vi "draw_spawn_positions.vi"(4 "error in":errorcluster, 7 "simx in":T1) -> (0 "error out":errorcluster, 3 "simx out":T1={"Config"={"Trajectory"={"Number of frames"=0, "Frame number"=0, "Trajectory"=""}, "Weather"={"id"=""}}, "Connections"={"Simulator Connection"=refnum, "server_ip"="127.0.0.1", "Port"=0, "Sensor connections"=[]}, "Map"={"lanes"={"x"=[], "y"=[], "z"=[]}, "StartPosition"={"start_points"={"locations"=[], "rotations"=[], "type"=[]}, "StartRotation"=[], "StartLocation"=[]}, "Draw Map Size"={"Width"=0, "Height"=0}, "DrawArea"={"min_Y"=0.0, "min_X"=0.0, "Scale X"=0.0, "Scale Y"=0.0}, "Map"=bytes[0], "Map Geojson"=""}})   [LabVIEW 2025]
doc: "Draw the possible spawn positions for the EGO vehicle on the map as dots. Adds the string \"Camera\" for the position where the camera is pointing (only on Editor mode)."
uses:
  controls/simx_connection.ctl
  controls/config.ctl
  controls/trajectory.ctl
  controls/weather.ctl
  controls/connections.ctl
  controls/start_points.ctl
  <vilib>/Utility/miscctls.llb/LVBoundsTypeDef.ctl
panel:
  out "Map":picture
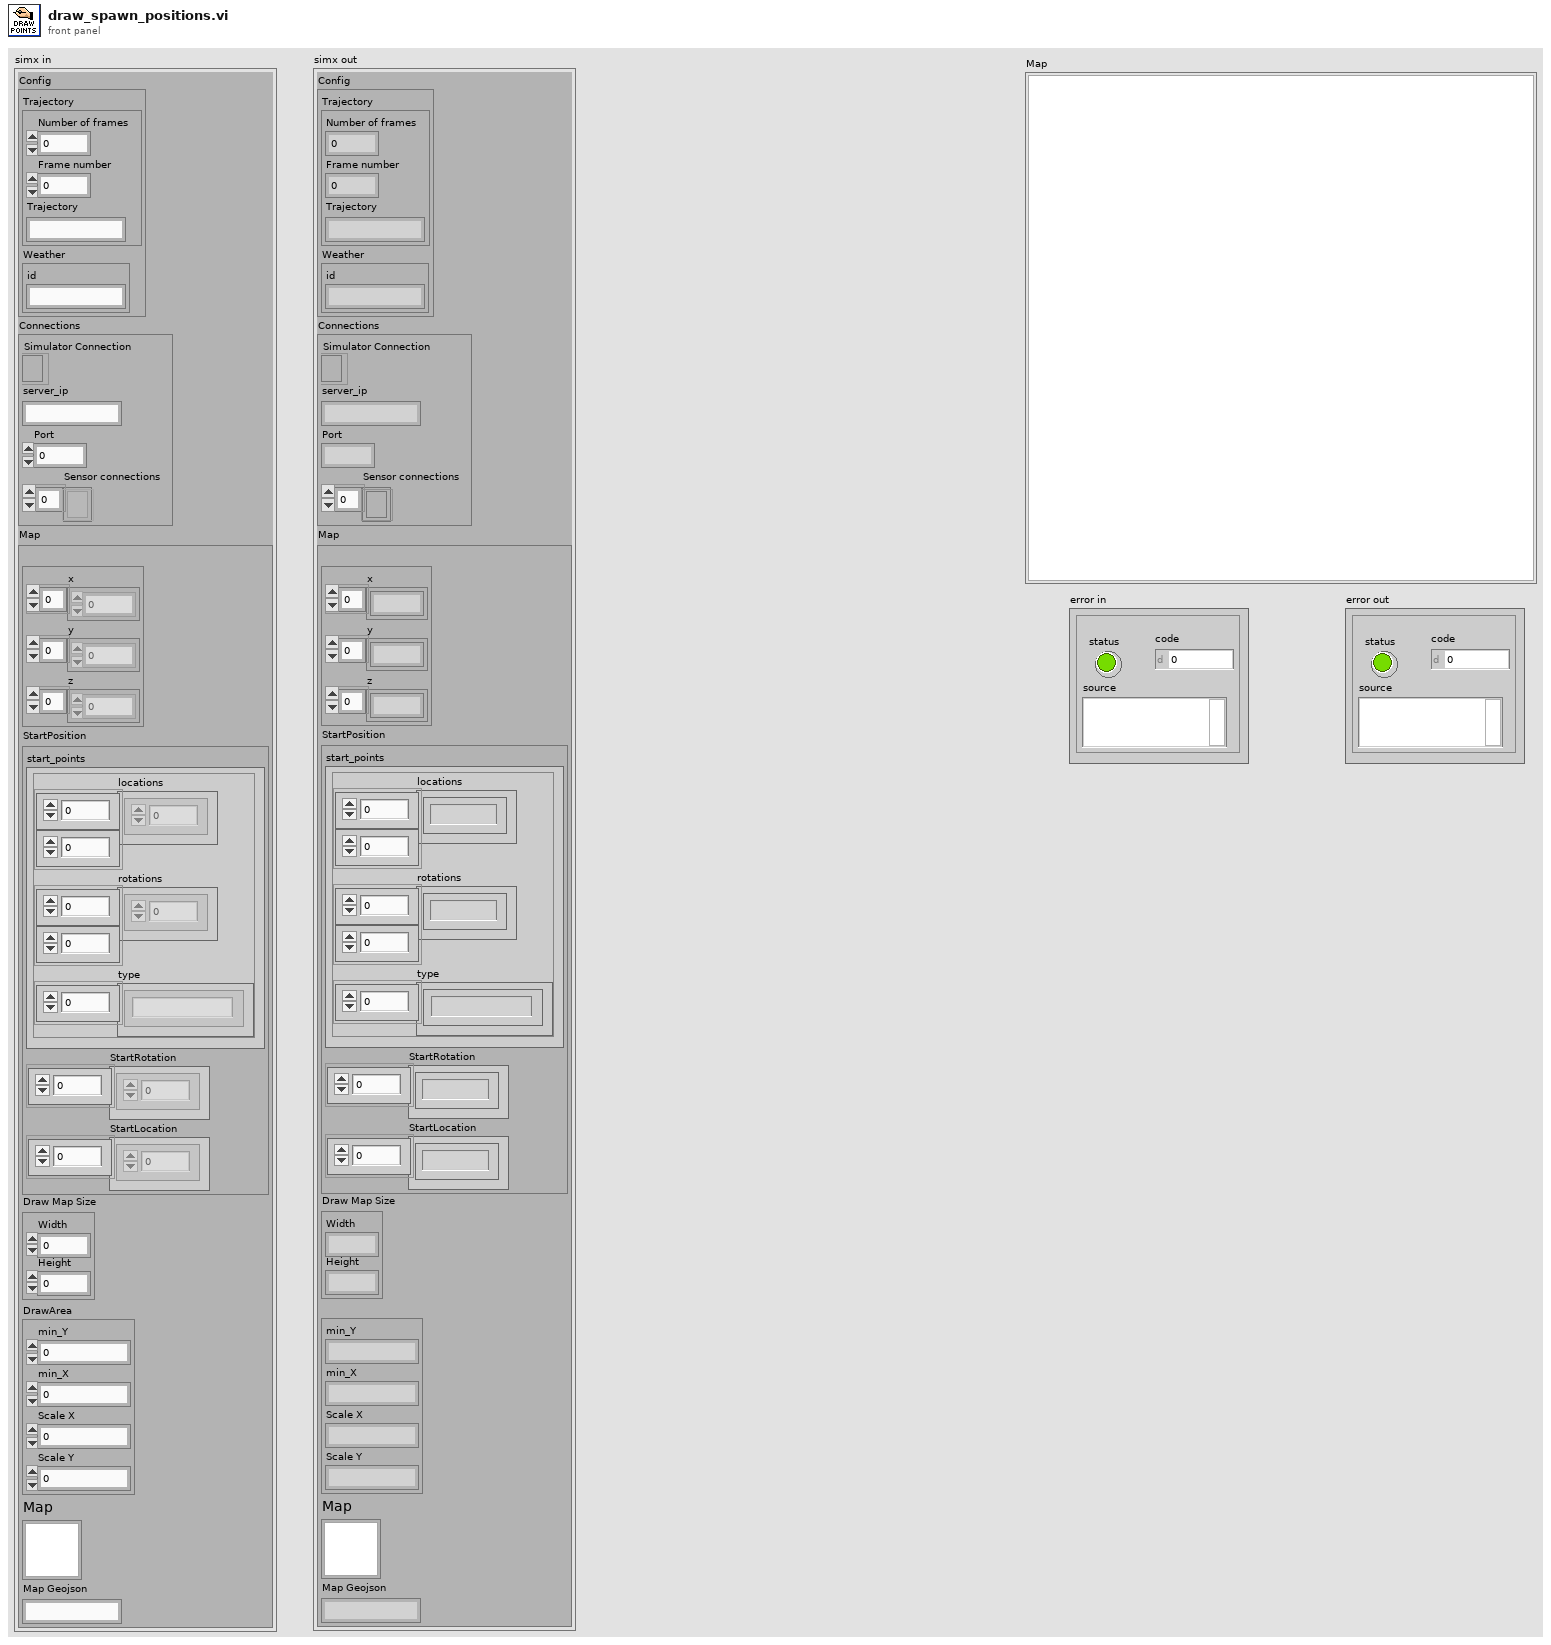
[diagram p1: front panel]
types:
  T1 = typedef "simx_connection.ctl" = cluster{"Config":T2, "Connections":T5, "Map":cluster{"lanes":cluster{"x":dbl[], "y":dbl[], "z":dbl[]}, "StartPosition":cluster{"start_points":T6, "StartRotation":dbl[], "StartLocation":dbl[]}, "Draw Map Size":T7, "DrawArea":cluster{"min_Y":dbl, "min_X":dbl, "Scale X":dbl, "Scale Y":dbl}, "Map":picture, "Map Geojson":string}}
  T2 = typedef "config.ctl" = cluster{"Trajectory":T3, "Weather":T4}
  T3 = typedef "trajectory.ctl" = cluster{"Number of frames":i32, "Frame number":i32, "Trajectory":string}
  T4 = typedef "weather.ctl" = cluster{"id":string}
  T5 = typedef "connections.ctl" = cluster{"Simulator Connection":refnum<k5>, "server_ip":string, "Port":i32, "Sensor connections":refnum<k5>[]}
  T6 = typedef "start_points.ctl" = cluster{"locations":dbl[][], "rotations":dbl[][], "type":string[]}
  T7 = typedef "LVBoundsTypeDef.ctl" = cluster{"Width":u32, "Height":u32}
  T8 = enum16{"User-specified Font", "Application Font", "System Font", "Dialog Font"}
  T9 = cluster{"horizontal":enum16{"left", "center", "right"}, "vertical":enum16{"top", "center", "bottom"}}
  T10 = cluster{"Font Name:":string, "Size":i16, "Strikeout?":bool, "Italic?":bool, "Underline?":bool, "Outline?":bool, "Shadow?":bool, "Bold?":bool}
  T11 = cluster{"Width":u16, "Style":enum32{"Solid", "Dash", "Dot", "DashDot", "DashDotDot"}}
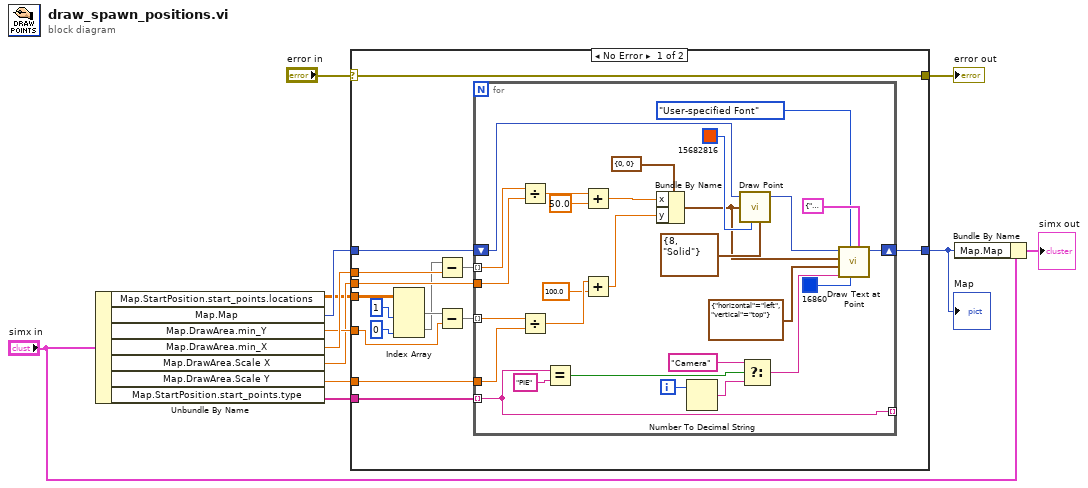
[diagram p0: block diagram]
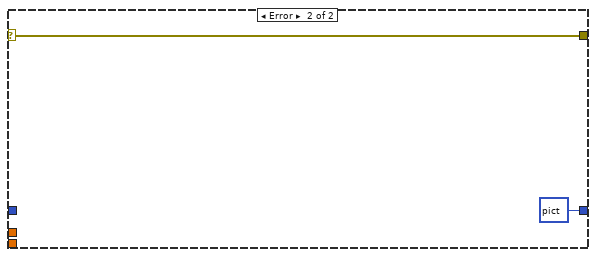
[diagram p2: hidden frame]
diagram:
  n1 = Unbundle By Name("simx in") -> ("Map.StartPosition.start_points.locations"=w1:dbl[][], "Map.Map"=w10:picture, "Map.DrawArea.min_Y"=w6:dbl, "Map.DrawArea.min_X"=w7:dbl, "Map.DrawArea.Scale X"=w5:dbl, "Map.DrawArea.Scale Y"=w4:dbl, "Map.StartPosition.start_points.type"=w3:string[])
  n2 = case shown="No Error" "error in" {
    selector: "error in" -> [w23 w57]
    tunnel: w1 -> [w24 _]
    tunnel: [w23 w57] -> w11
    tunnel: w10 -> [w22 _]
    tunnel: [w21 picture data[5B] ("Map")] -> w9
    tunnel: w7 -> [w20 _]
    tunnel: w6 -> [w19 _]
    tunnel: w5 -> [w18 _]
    tunnel: w4 -> [w17 _]
    tunnel: w3 -> [w13 _]
    frame No Error {
      n3 = Index Array(array=w24, index (col) #1=1 ("disabled index (col)"), index (col) #2=0 ("index (col)")) -> (element #1=w25:dbl[], element #2=w16:dbl[])  [unwired: 2 in]
      n4 = Subtract(x=w16, y=w20) -> (x-y=w14:dbl[])
      n5 = Subtract(x=w25, y=w19) -> (x-y=w15:dbl[])
      n6 = for {
        shift-right: [w50] -> w21
        shift-left: w22 -> [w54]
        tunnel: w18 -> [w43]
        tunnel: w17 -> [w42]
        tunnel: w15 -> [w40] mode=indexing
        tunnel: w14 -> [w41] mode=indexing
        tunnel: [w33] -> _ mode=indexing
        tunnel: w13 -> [w33] mode=indexing
        i -> [w48]
        n7 = Divide(x=w41, y=w43) -> (x/y=w39:dbl)
        n8 = Divide(x=w40, y=w42) -> (x/y=w38:dbl)
        n9 = Equal?(x=w33, y="PIE") -> (x = y?=w34:bool)
        n10 = Add(x=w39, y=50.0) -> (x+y=w37:dbl)
        n11 = Add(x=w38, y=100.0) -> (x+y=w36:dbl)
        n12 = Bundle By Name(cluster=cluster{"x":i16, "y":i16} {"x"=0, "y"=0} ("point(x,y)"), "x"=w37, "y"=w36) -> (w49:cluster{"x":i16, "y":i16})
        n13 = Number To Decimal String(number=w48) -> (decimal integer string=w30:string)  [unwired: 1 in]
        n14 = call <vilib>:"Draw Point.vi"("picture"=w54, "point(x,y)"=w49, "color(black)"=u32 15682816, "pen"=T11 {"Width"=8, "Style"=enum."Solid"}) -> ("new picture"=w55:picture)  [unwired: 5 in]
        n15 = Select(t="Camera" ("y"), s=w34, f=w30) -> (s? t:f=w29:string)
        n16 = call <vilib>:"Draw Text at Point.vi"("[user-specified font]"=T10 {"Font Name:"="Application Font", "Size"=40, "Strikeout?"=FALSE, "Italic?"=FALSE, "Underline?"=FALSE, "Outline?"=FALSE, "Shadow?"=FALSE, "Bold?"=TRUE}, "text color(black)"=u32 16860, "desired font(Application)"=T8."User-specified Font", "text"=w29, "alignment(left, top)"=T9 {"horizontal"=enum."left", "vertical"=enum."top"}, "origin"=w49, "picture"=w55) -> ("new picture"=w50:picture)  [unwired: 3 in, 1 out]
      }
    }
    frame Error {
    }
  }
  "error out" <- w11
  "Map" <- w9
  n17 = Bundle By Name(cluster="simx in", "Map.Map"=w9) -> (→"simx out":T1)
